vi "Get Department.vi"(8 "error in (no error)":errorcluster caption="错误输入（无错误）", 11 "Access Department 输入":refnum<class "Access Department.lvclass">) -> (0 "error out":errorcluster caption="错误输出", 2 "字符串":string, 3 "Access Department 输出":refnum<class "Access Department.lvclass">)   [LabVIEW 2017, in "Access Department.lvclass"]
uses:
  Access Department.lvclass
  Abstract Department/Abstract Department.lvclass
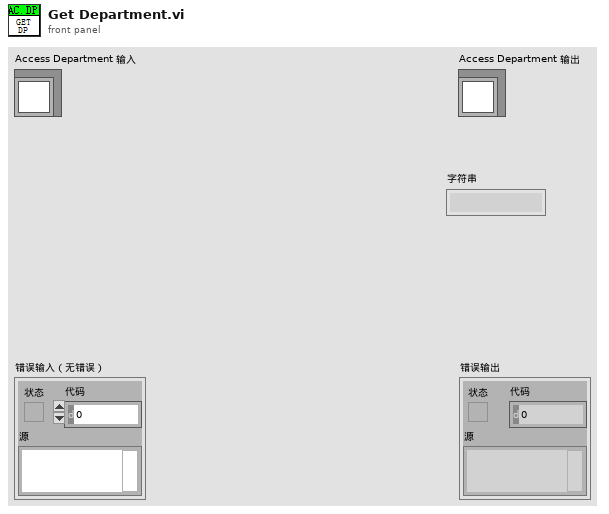
[diagram p1: front panel]
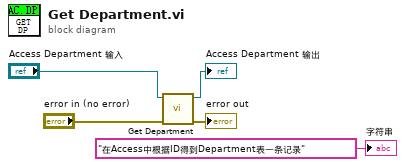
[diagram p0: block diagram]
diagram:
  n1 = call-parent "Get Department.vi"("error in (no error)"="error in (no error)", "Abstract Department 输入"="Access Department 输入") -> ("error out"=→"error out":errorcluster, "Abstract Department 输出"=→"Access Department 输出":refnum<class "Access Department.lvclass">)  [unwired: 7 in, 1 out]
  "字符串" <- "在Access中根据ID得到Department表一条记录" ("字符串")
